vi "Select Command.vi"(10 "Host LCD Command":T1, 11 "FPGA LCD Command":T1) -> (1 "operation":u32, 2 "device index":i8, 3 "FPGA? True : False":bool)   [LabVIEW 2017, in "HD44780 FPGA.lvlib"]
uses:
  HD44780 FPGA.lvlib
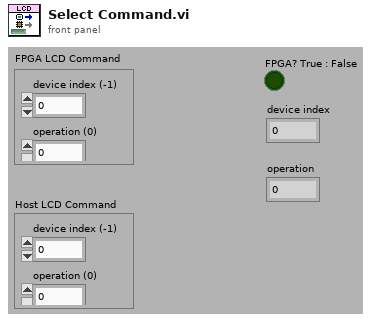
[diagram p1: front panel]
types:
  T1 = cluster{"device index (-1)":i8, "operation (0)":u32}
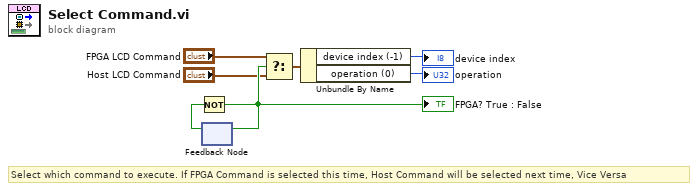
[diagram p0: block diagram]
diagram:
  # "Select which command to execute. If FPGA Command is selected this time, Host Command will be selected next time, Vice Versa"
  n1 = feedback #1() -> (w7:bool)  [unwired: 1 in]
  n2 = Not(x=w7) -> (.not. x?=w6:bool)
  "FPGA? True : False" <- w6
  n3 = feedback-in #1(w6) -> ()
  n4 = Select(t="FPGA LCD Command", s=w6, f="Host LCD Command") -> (s? t:f=w3:T1)
  n5 = Unbundle By Name(w3) -> ("device index (-1)"=→"device index":i8, "operation (0)"=→"operation":u32)
